vi "Airmass.vi"(1 "temps sidéral":dbl format="%<%H:%M:%S>t", 2 "DEC":string, 3 "RA":string) -> (0 "airmass":dbl format="%.3g")   [LabVIEW 2019]
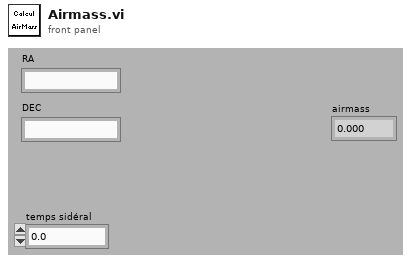
[diagram p1: front panel]
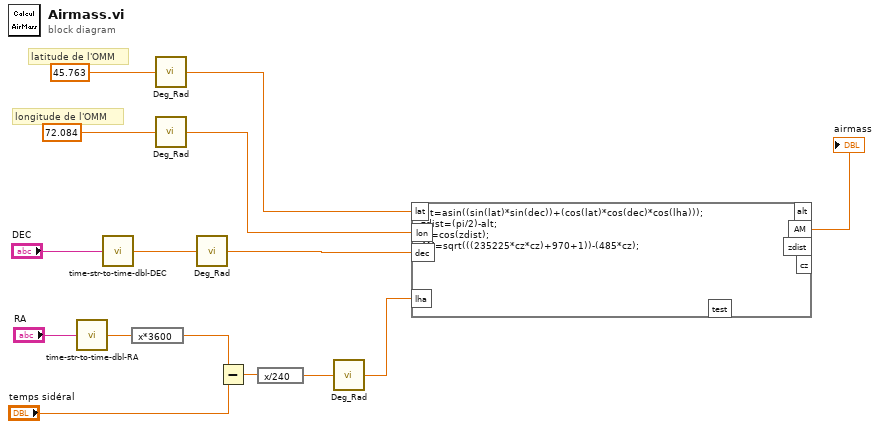
[diagram p0: block diagram]
diagram:
  # "longitude de l'OMM"
  # "latitude de l'OMM"
  n1 = call "time-str-to-time-dbl-RA.vi"("Chaîne"="RA") -> ("TCS_coords"=w5:dbl)
  n2 = call "time-str-to-time-dbl-DEC.vi"("Chaîne"="DEC") -> ("TCS_coords"=w3:dbl)
  n3 = expression code="x*3600"(w5) -> (w7:dbl)
  n4 = call "Deg_Rad.vi"("Angle"=45.763) -> ("RadRot"=w14:dbl)
  n5 = call "Deg_Rad.vi"("Angle"=72.084) -> ("RadRot"=w15:dbl)
  n6 = call "Deg_Rad.vi"("Angle"=w3) -> ("RadRot"=w13:dbl)
  n7 = Subtract(x=w7, y="temps sidéral") -> (x-y=w2:dbl)
  n8 = expression code="x/240"(w2) -> (w1:dbl)
  n9 = call "Deg_Rad.vi"("Angle"=w1) -> ("RadRot"=w12:dbl)
  n10 = formula code="alt=asin((sin(lat)*sin(dec))+(cos(lat)*cos(dec)*cos(lha)));\nzdist=(pi/2)-alt;\ncz=cos(zdist);\nAM=sqrt(((235225*cz*cz)+970+1))-(485*cz);"("lat"=w14, "lon"=w15, "dec"=w13, "lha"=w12) -> ("AM"=→"airmass":dbl)  [unwired: 4 out]
